vi "Convert Callback To Dbl Click.vi"(6 "Return Meet Filter Selection":bool=TRUE, 8 "error in":errorcluster, 10 "Data":variant, 11 "SystemDefinitionBrowser Ref":T2) -> (0 "error out":errorcluster, 2 "Valid?":bool, 3 "Dbl Clicked Item":T1)   [LabVIEW 2020, in "NI_VS UI System Tree.lvlib"]
uses:
  <vilib>/NI VeriStand/UI Controls/System Definition Tree/NI_VS UI System Tree.lvlib
  <vilib>/NI VeriStand/UI Controls/System Definition Tree/System Definition Tree Ref.ctl
  NationalInstruments.VeriStand.SystemStorageUI
  <vilib>/NI VeriStand/UI Controls/System Definition Tree/Node Ref.ctl
  NationalInstruments.VeriStand.SystemStorage
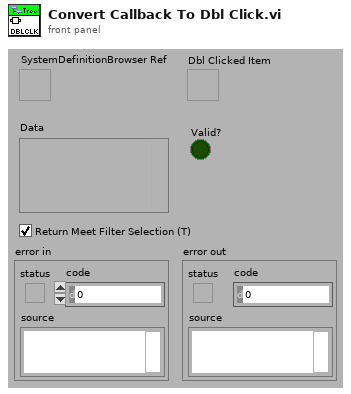
[diagram p1: front panel]
types:
  T1 = typedef "NI_VS UI System Tree.lvlib/Node Ref.ctl" = refnum<k24>
  T2 = typedef "NI_VS UI System Tree.lvlib/System Definition Tree Ref.ctl" = refnum<k24>
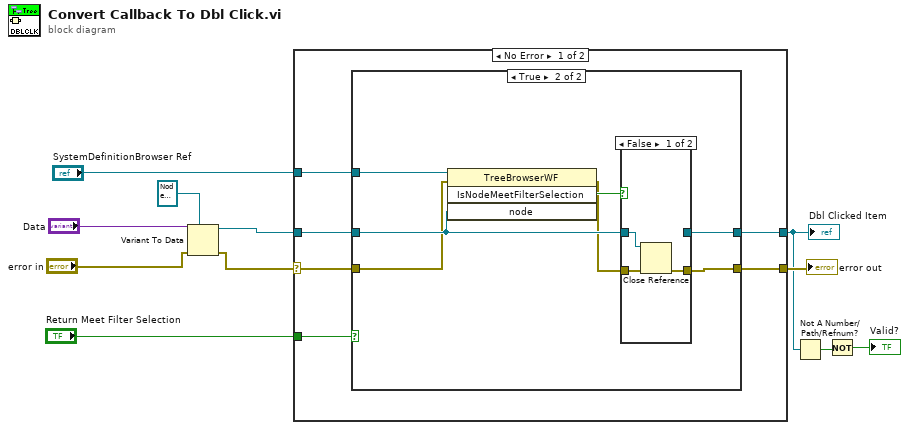
[diagram p0: block diagram]
diagram:
  n1 = Variant To Data(error in="error in", type=T1 refnum ("Selected Item"), Variant="Data") -> (data=w7:T1, error out=w9:errorcluster)
  n2 = case shown="No Error" w9 {
    selector: w9 -> [w14 w32]
    tunnel: "SystemDefinitionBrowser Ref" -> [w17 _]
    tunnel: w7 -> [w15 _]
    tunnel: "Return Meet Filter Selection" -> [w16 _]
    tunnel: [w13 w32] -> w5
    tunnel: [w12 _] -> w3
    frame No Error {
      n3 = case shown="True" w16 {
        tunnel: w17 -> [_ w26]
        tunnel: w15 -> [w18 w25]
        tunnel: w14 -> [w19 w24]
        tunnel: [w19 w23] -> w13
        tunnel: [w18 w20] -> w12
        frame False {
        }
        frame True {
          n4 = invoke class="TreeBrowserWF" method="IsNodeMeetFilterSelection"(reference=w26, error in=w24, "node"=w25) -> (error out=w21:errorcluster, "IsNodeMeetFilterSelection"=w22:bool)  [unwired: 1 in, 2 out]
          n5 = case shown="False" w22 {
            tunnel: w25 -> [w29 w30]
            tunnel: w21 -> [w28 w31]
            tunnel: [w27 w31] -> w23
            tunnel: [_ w30] -> w20
            frame False {
              n6 = Close Reference(reference=w29, error in (no error)=w28) -> (error out=w27:errorcluster)
            }
            frame True {
            }
          }
        }
      }
    }
    frame Error {
    }
  }
  "error out" <- w5
  "Dbl Clicked Item" <- w3
  n7 = Not A Number/Path/Refnum?(number/path/refnum=w3) -> (NaN/Path/Refnum?=w2:bool)
  n8 = Not(x=w2) -> (.not. x?=→"Valid?":bool)
